vi "Write.vi"(8 "error in (no error)":errorcluster, 10 "String":string, 11 "String in":refnum<class "String.lvclass">) -> (0 "error out":errorcluster, 3 "String out":refnum<class "String.lvclass">)   [LabVIEW 2021, in "Variable.lvlib" / "String.lvclass"]
uses:
  String.lvclass
  String.lvclass/String.ctl
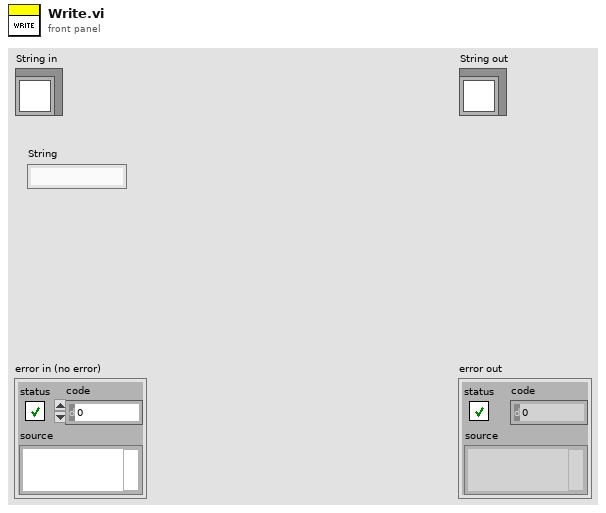
[diagram p1: front panel]
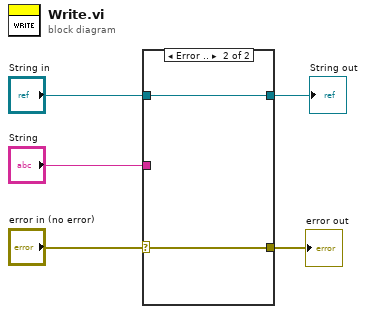
[diagram p0: block diagram]
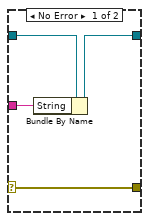
[diagram p2: hidden frame]
diagram:
  n1 = case shown="Error .." "error in (no error)" {
    selector: "error in (no error)" -> [w6 w10]
    tunnel: "String in" -> [w9 w11]
    tunnel: [w8 w11] -> w4
    tunnel: "String" -> [w7 _]
    tunnel: [w6 w10] -> w1
    frame No Error {
      n2 = Bundle By Name(cluster=w9, "String"=w7) -> (w8:refnum<class "String.lvclass">)
    }
    frame Error {
    }
  }
  "error out" <- w1
  "String out" <- w4
